vi "Convert PID Gains (PI).vi"(0 "proportional":sgl, 1 "gains pattern (Parallel)":T3=1 items=["Academic", "Parallel", "Series"], 5 "integral":sgl, 9 "sampling time":sgl min=0, 11 "error in (no error)":errorcluster, 12 "proportional unit (Gain (K))":T2 items=["Gain (K)", "Band (PB)"], 13 "integral unit (Hz)":T1 items=["Hz", "s", "min"]) -> (4 "gains":T4 {"proportional gain" step=0.125}, 15 "error out":errorcluster)   [LabVIEW 2020]
doc: "Converts PID gains in the Academic, Parallel, or Series form to the normalized Parallel form that the PID VI expects."
uses:
  <vilib>/rvi/Analysis/control/PID/Typedef/niFpgaPID_PIGains.ctl
  <vilib>/rvi/Analysis/host/Private/PID Gains Pattern.ctl
  <vilib>/rvi/Analysis/host/Private/PID Proportional Unit.ctl
  <vilib>/rvi/Analysis/host/Private/PID Integral Derivative Unit.ctl
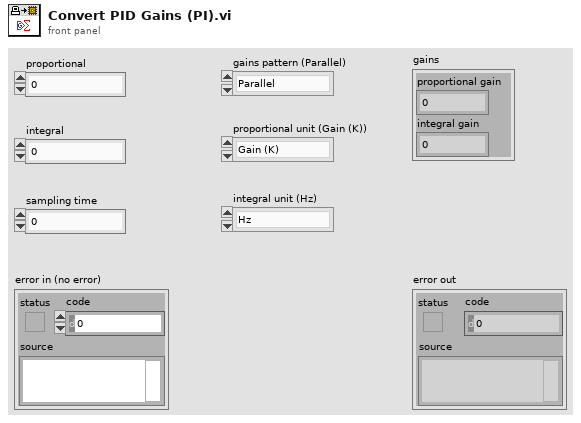
[diagram p1: front panel]
types:
  T1 = typedef "PID Integral Derivative Unit.ctl" = u8
  T2 = typedef "PID Proportional Unit.ctl" = u8
  T3 = typedef "PID Gains Pattern.ctl" = u8
  T4 = typedef "niFpgaPID_PIGains.ctl" = cluster{"proportional gain":sgl, "integral gain":sgl}
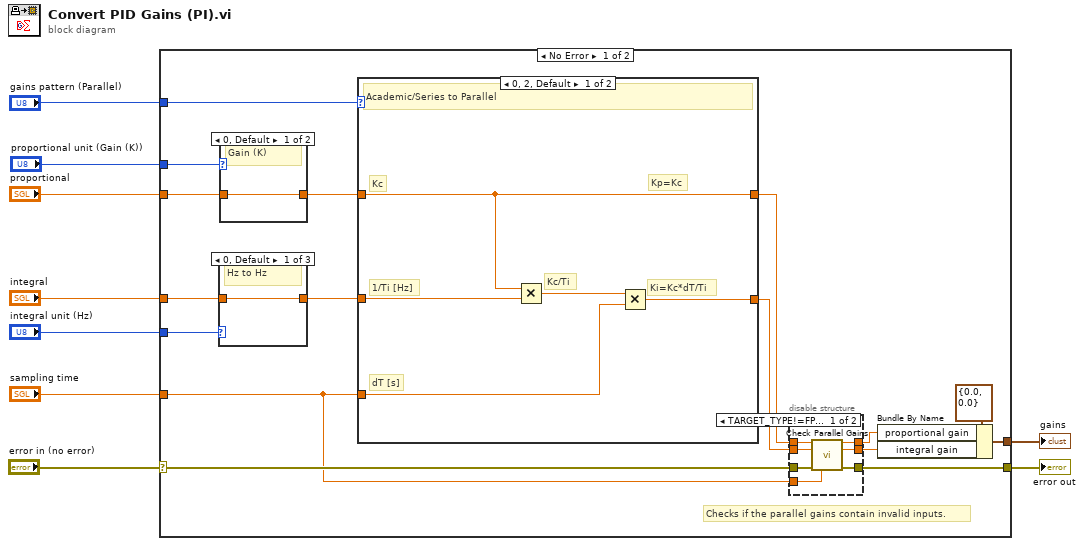
[diagram p0: block diagram]
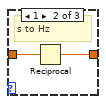
[diagram p3: hidden frame]
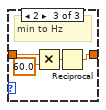
[diagram p4: hidden frame]
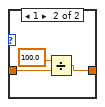
[diagram p5: hidden frame]
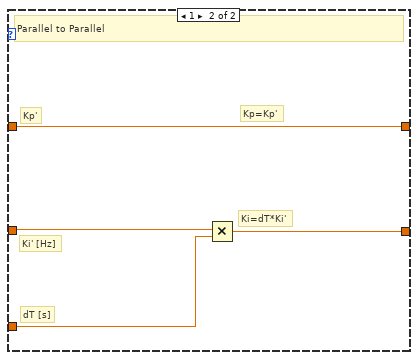
[diagram p6: hidden frame]
diagram:
  n1 = case shown="No Error" "error in (no error)" {
    selector: "error in (no error)" -> [w23 w56]
    tunnel: "gains pattern (Parallel)" -> [w25 _]
    tunnel: "sampling time" -> [w10 _]
    tunnel: [w24 w56] -> w7
    tunnel: "proportional" -> [w19 _]
    tunnel: "proportional unit (Gain (K))" -> [w18 _]
    tunnel: "integral" -> [w16 _]
    tunnel: "integral unit (Hz)" -> [w15 _]
    tunnel: [w13 _] -> w4
    frame No Error {
      # "Checks if the parallel gains contain invalid inputs."
      n2 = case shown="0, Default" w15 {
        tunnel: w16 -> [w36 w37 w41]
        tunnel: [w36 w38 w39] -> w17
        frame 0, Default {
          # "Hz to Hz"
        }
        frame 1 {
          # "s to Hz"
          n3 = Reciprocal(x=w37) -> (1/x=w38:sgl)
        }
        frame 2 {
          # "min to Hz"
          n4 = Multiply(x=w41, y=sgl 60.0) -> (x*y=w42:sgl)
          n5 = Reciprocal(x=w42) -> (1/x=w39:sgl)
        }
      }
      n6 = case shown="0, Default" w18 {
        tunnel: w19 -> [w43 w44]
        tunnel: [w43 w46] -> w20
        frame 0, Default {
          # "Gain (K)"
        }
        frame 1 {
          n7 = Divide(x=sgl 100.0, y=w44) -> (x/y=w46:sgl)
        }
      }
      n8 = case shown="0, 2, Default" w25 {
        tunnel: w20 -> [w49 w55]
        tunnel: w17 -> [w48 w53]
        tunnel: w10 -> [w47 w52]
        tunnel: [w49 w55] -> w22
        tunnel: [w50 w54] -> w21
        frame 0, 2, Default {
          # "Kp=Kc"
          # "Ki=Kc*dT/Ti"
          # "Kc/Ti"
          # "dT [s]"
          # "Kc"
          # "1/Ti [Hz]"
          # "Academic/Series to Parallel"
          n9 = Multiply(x=w49, y=w48) -> (x*y=w51:sgl)
          n10 = Multiply(x=w51, y=w47) -> (x*y=w50:sgl)
        }
        frame 1 {
          # "Kp=Kp'"
          # "dT [s]"
          # "Ki=dT*Ki'"
          # "Kp'"
          # "Ki' [Hz]"
          # "Parallel to Parallel"
          n11 = Multiply(x=w53, y=w52) -> (x*y=w54:sgl)
        }
      }
      n12 = disable-structure shown="TARGET_TYPE!=FPGA, Default" {
        disable-tunnel: [w32 w35] -> w24
        disable-tunnel: w23 -> [w31 w35]
        disable-tunnel: w22 -> [w30 w34]
        disable-tunnel: w21 -> [w29 w33]
        disable-tunnel: [w28 w34] -> w12
        disable-tunnel: [w27 w33] -> w11
        disable-tunnel: w10 -> [w26 _]
        frame condition #0 (active) {
          n13 = call <vilib>:"Check Parallel Gains.vi"("proportional gain in"=w30, "integral gain in (0)"=w29, "error in (no error)"=w31, "sampling time"=w26) -> ("proportional gain out"=w28:sgl, "integral gain out"=w27:sgl, "error out"=w32:errorcluster)  [unwired: 7 in, 2 out]
        }
        frame condition #1 {
        }
      }
      n14 = Bundle By Name(cluster=T4 {"proportional gain"=0.0, "integral gain"=0.0} ("gains"), "proportional gain"=w12, "integral gain"=w11) -> (w13:T4)
    }
    frame Error {
    }
  }
  "error out" <- w7
  "gains" <- w4
